vi "Set LVRT Module Path.vi"(8 "error in":errorcluster, 11 "Module Path":string) -> (0 "error out":errorcluster)   [LabVIEW 2019, in "grpc-lvsupport.lvlib"]
uses:
  grpc-lvsupport.lvlib
  <vilib>/Utility/error.llb/Error Cluster From Error Code.vi
  <vilib>/Utility/error.llb/Simple Error Handler.vi
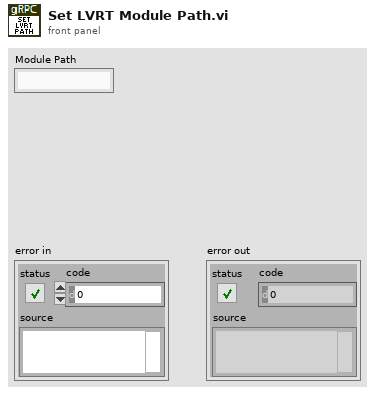
[diagram p1: front panel]
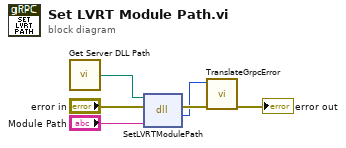
[diagram p0: block diagram]
diagram:
  n1 = call "Get Server DLL Path.vi"() -> ("Server dll path"=w4:path)
  n2 = dll-call lib="?" fn="SetLVRTModulePath"(path in=w4, error in="error in", "modulePath"="Module Path") -> (error out=w5:errorcluster, "return type"=w1:i32)  [unwired: 2 in, 1 out]
  n3 = call "TranslateGrpcError.vi"("error in"=w5, "Error Code"=w1) -> ("error out"=→"error out":errorcluster)  [unwired: 9 in]
